vi "Commit Transaction.vi"(8 "error in":errorcluster, 11 "DB-Interface in":refnum<class "DB-Interface.lvclass">) -> (0 "error out":errorcluster, 3 "DB-Interface out":refnum<class "DB-Interface.lvclass">)   [LabVIEW 2022 SP3, in "hse-db.lvlib" / "DB-Interface.lvclass"]
doc: "Commit a transaction. Either all SQL-commands get commited or, in case of an error, all get rejected.\n\n____\nHAMPEL SOFTWARE ENGINEERING v1.4.0 (2023-12-19 09:52)"
uses:
  DB-Interface.lvclass
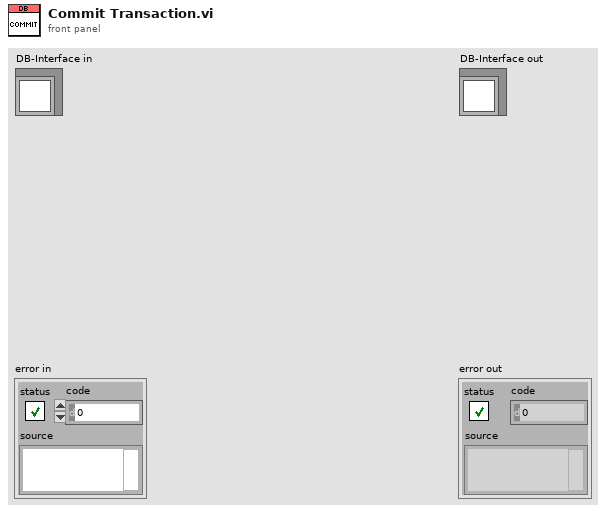
[diagram p1: front panel]
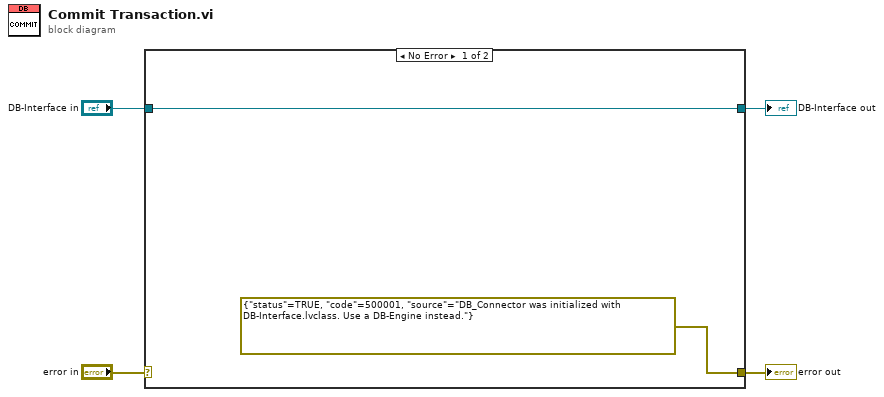
[diagram p0: block diagram]
diagram:
  n1 = case shown="No Error" "error in" {
    selector: "error in" -> [_ w8]
    tunnel: [errorcluster {"status"=TRUE, "code"=500001, "source"="DB_Connector was initialized with DB-Interface.lvclass. Use a DB-Engine instead."} ("error IO") w8] -> w3
    tunnel: [w6 w7] -> w1
    tunnel: "DB-Interface in" -> [w6 w7]
    frame No Error {
    }
    frame Error {
    }
  }
  "error out" <- w3
  "DB-Interface out" <- w1
